vi "Close.vi"(8 "error in (no error)":errorcluster, 11 "AcPwrSimBase in":refnum<class "AcPwrSimBase.lvclass">) -> (0 "error out":errorcluster, 3 "AcPwrSimBase out":refnum<class "AcPwrSimBase.lvclass">)   [LabVIEW 2018, in "AcPwrPlugins.lvlib" / "AcPwrSimBase.lvclass"]
doc: "This VI closes the reference to the instrument(s)."
uses:
  AcPwrSimBase.lvclass
  Database/DatabaseBaseClass/DatabaseBaseClass.lvclass
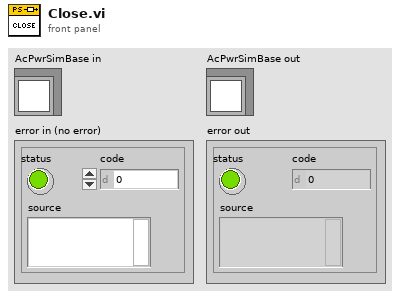
[diagram p1: front panel]
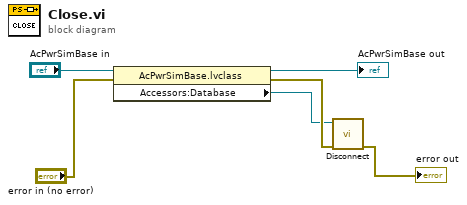
[diagram p0: block diagram]
diagram:
  n1 = property class="AcPwrSimBase.lvclass"(reference="AcPwrSimBase in", error in="error in (no error)") -> (reference out=→"AcPwrSimBase out":refnum<class "AcPwrSimBase.lvclass">, error out=w2:errorcluster, "Accessors:Database"=w1:refnum<class "DatabaseBaseClass.lvclass">)
  n2 = call-dynamic "Disconnect.vi"("error in (no error)"=w2, "DatabaseBaseClass in"=w1) -> ("error out"=→"error out":errorcluster)  [unwired: 8 in, 1 out]
